vi "field_sweep_agilent_0.vi"() -> ()   [LabVIEW 2016]
uses:
  Controls/Data.ctl
  Controls/State.ctl
  <vilib>/Utility/error.llb/DialogType.ctl
  <vilib>/DAQmx/write.llb/DAQmx Write (Analog DBL 1Chan 1Samp).vi
  <vilib>/DAQmx/create/channels.llb/DAQmx Create Channel (AO-Voltage-Basic).vi
  <vilib>/DAQmx/miscellaneous.llb/DAQmx Fill In Error Info.vi
  <instrlib>/Keysight PNA Series/Keysight PNA Series.lvlib
panel:
  in  "Display Format":i32(ring) items=["Magnitude Linear", "Magnitude Logarithmic", "Phase", "Unwrapped phase", "Imaginary", "Real", "Polar", "Smith Chart", "Smith Admittance", "SWR", "Group Delay", "Kelvin", "Fahrenheit", "Celsius"]
  in  "Data Type":i32(ring) items=["FDATA", "RDATA", "SDATA", "FMEM", "SMEM", "SDIV"]
  in  "Sweep Generation":i32(ring)=1 items=["Stepped", "Analog"]
  in  "IF Bandwidth (Hz)":dbl=1000.0 min=1.0 max=40000.0 step=1.0 format="%#_6p"
  in  "Sweep Mode":i32(ring) items=["Chopped", "Alternate"]
  in  "Sweep Type":i32(ring) items=["Linear", "Logarithmic", "Power", "CW", "Segment", "Phase"]
  out "Analyzer Name Out":refnum<visa-resource-name>
  in  "Analyzer name In":refnum<visa-resource-name>="vna"
  in  "Clear button":bool
  in  "Hysteresis":bool caption="Hysteresis On/Off"
  out "DAQ channel Out":tag="DAQ_6363/ao1"
  in  "Averaging Points":i32=10 min=1 max=3201 step=1
  in  "DAQ channel In":tag="DAQ_6363/ao1"
  in  "Exit Button":bool
  in  "Speed (Oe/sec)":dbl=5.0
  in  "Frequency (Hz)":dbl=3000000000.0 min=10000000.0 max=6000000000.0 format="%#_6p"
  in  "Save Button":bool
  out "Status":string="Initializing..."
  out "Cursor":cluster{"x":dbl, "y":dbl} {"x" format="%.2f"; "y" format="%.5f"}
  out "Error Out":errorcluster={"status"=TRUE, "code"=-1073807346, "source"="VISA Open in Keysight PNA Series.lvlib:Initialize.vi->field_sweep_agilent.vi"}
  in  "Error In (no error)":errorcluster
  out "SpectrumGraph":cluster{"Old Field":dbl[], "Old Signal":dbl[]}[](graph)
  in  "S-parameter":i32(ring)=1 caption="Measurement" items=["S11", "S21"]
  in  "Start Button":bool
  in  "Stop Button":bool
  in  "Output Power (dBm)":dbl=1.0 min=-25.0 max=20.0 step=0.5
  in  "Number of Points":i32=1000 min=1 max=3201 step=1
  in  "Stop H Field (Oe)":dbl=1500.0 min=-6000.0 max=6000.0 format="%#_6f"
  in  "Start H Field (Oe)":dbl=1000.0 min=-6000.0 max=6000.0 format="%#_6f"
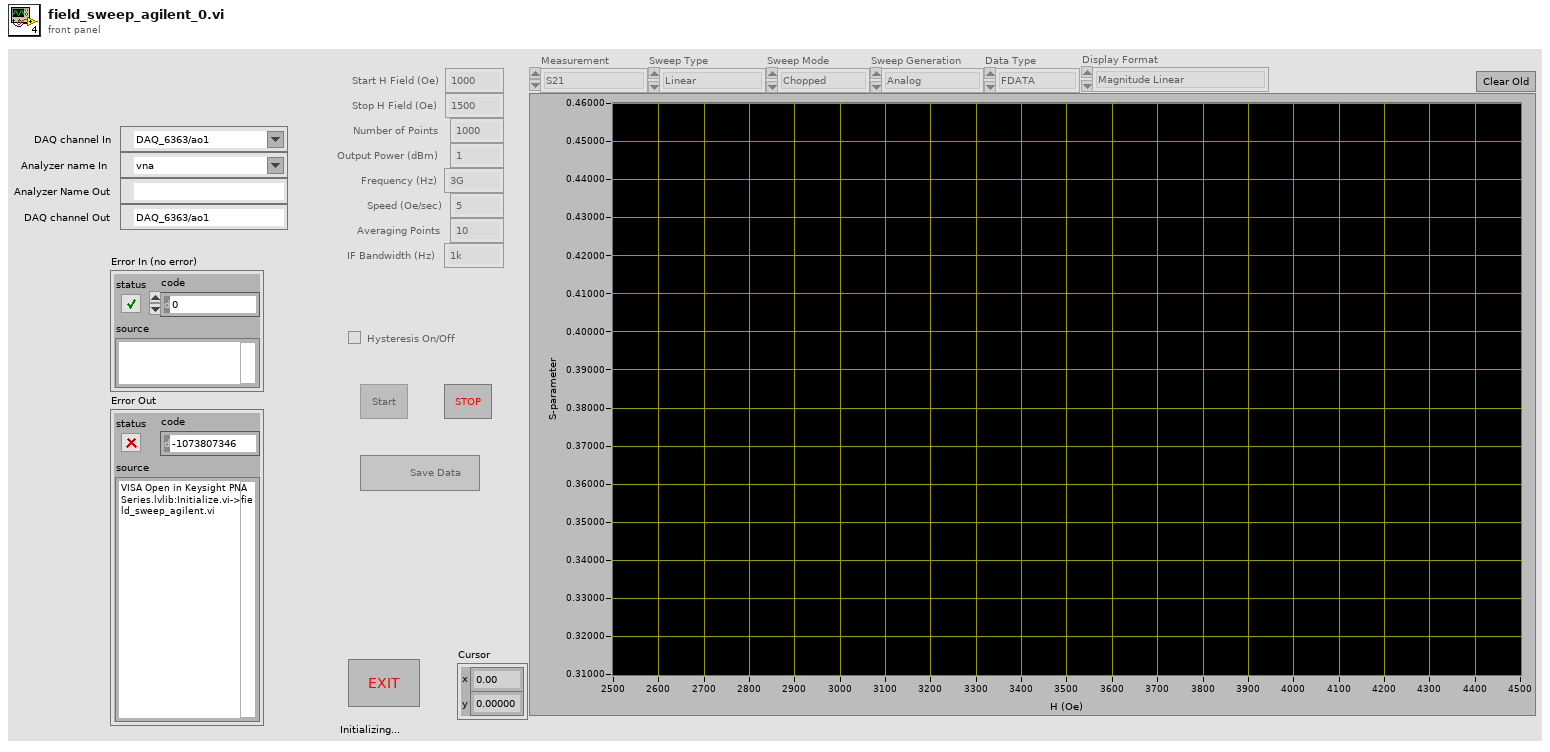
[diagram p1: front panel]
types:
  T1 = typedef "State.ctl" = enum16{"Init", "Idle", "Sweeping up", "Sweeping down", "Running", "Running first time", "Running down", "Shutdown"}
  T2 = typedef "Data.ctl" = cluster{"Field":dbl[], "Signal":dbl[], "Old Field":dbl[], "Old Signal":dbl[]}
  T3 = typedef "DialogType.ctl" = u16
  T4 = typedef "LVPoint32TypeDef.ctl" = cluster{"Horizontal":i32, "Vertical":i32}
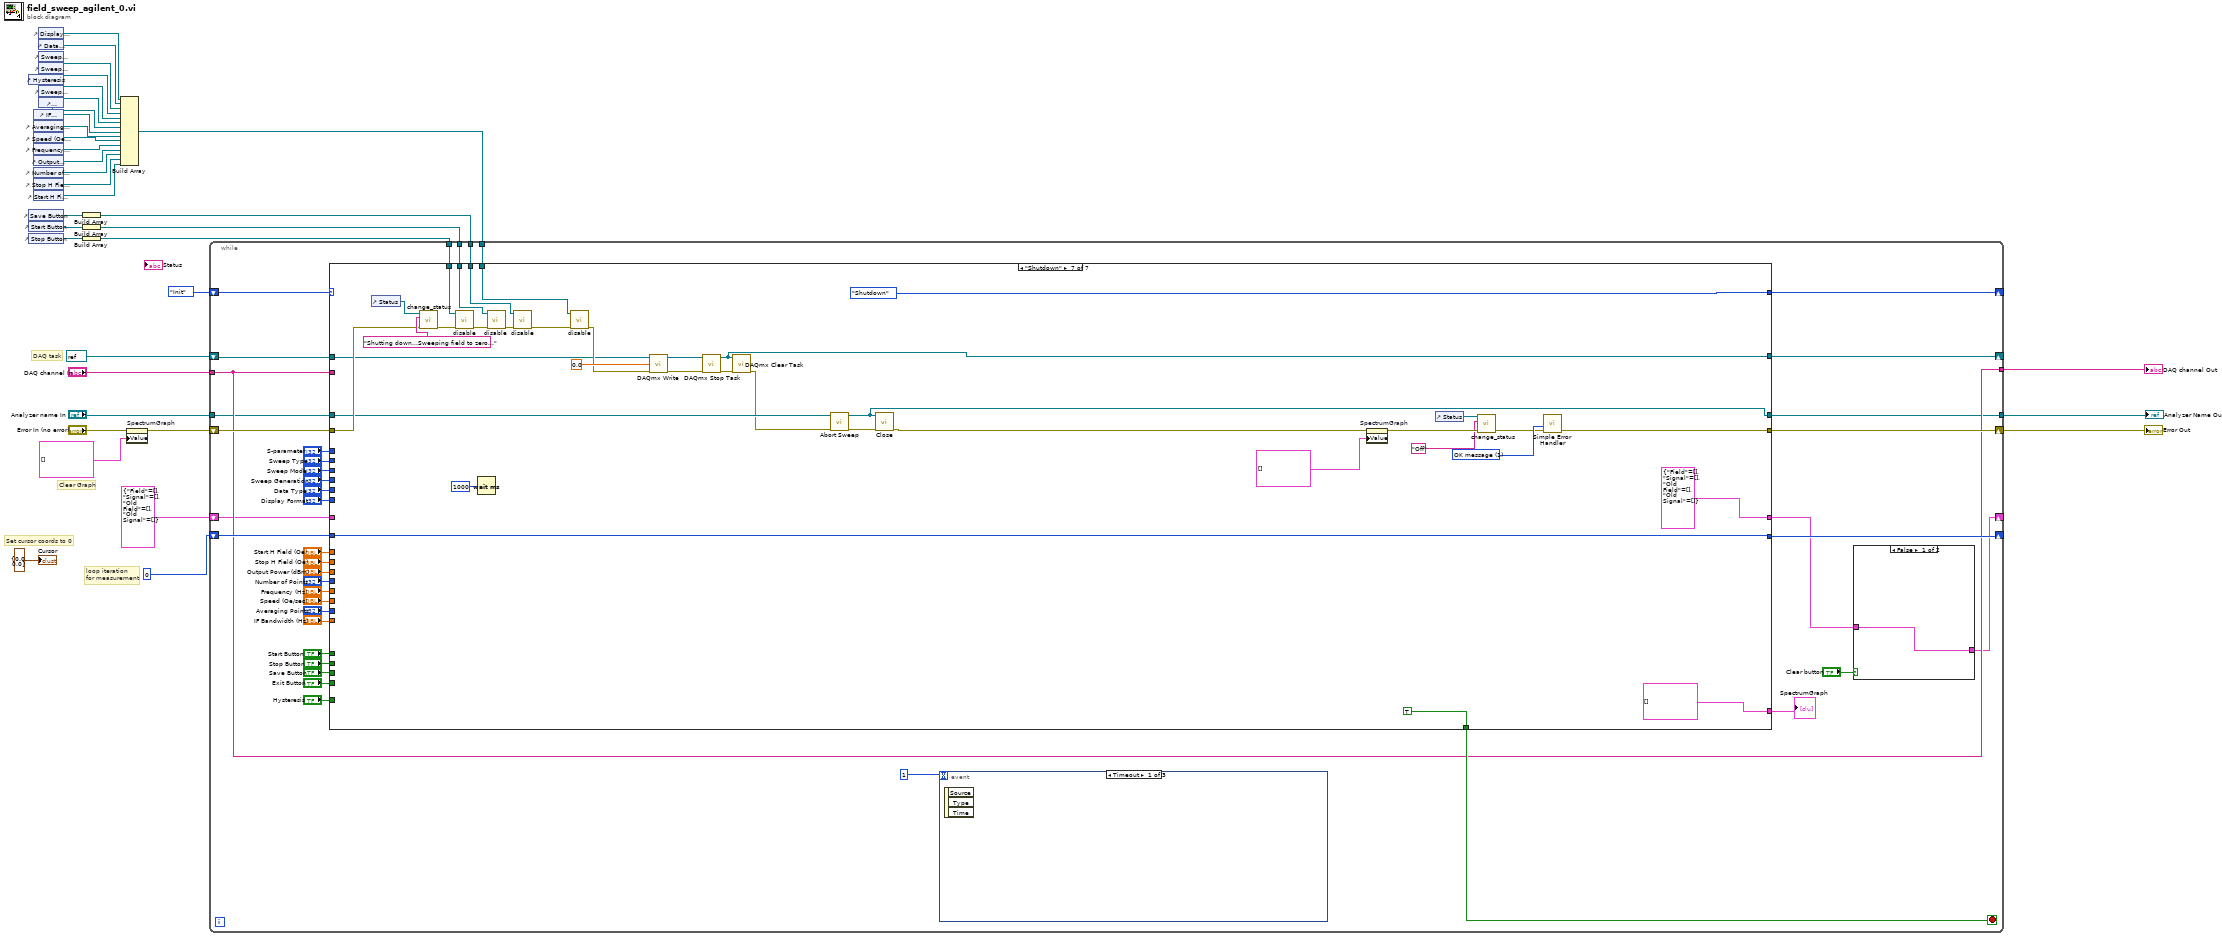
[diagram p0: block diagram]
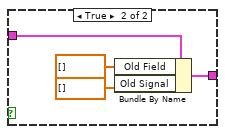
[diagram p2: hidden frame]
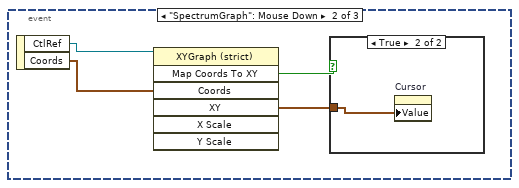
[diagram p3: hidden frame]
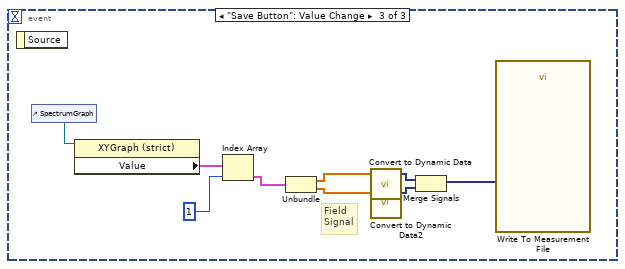
[diagram p5: hidden frame]
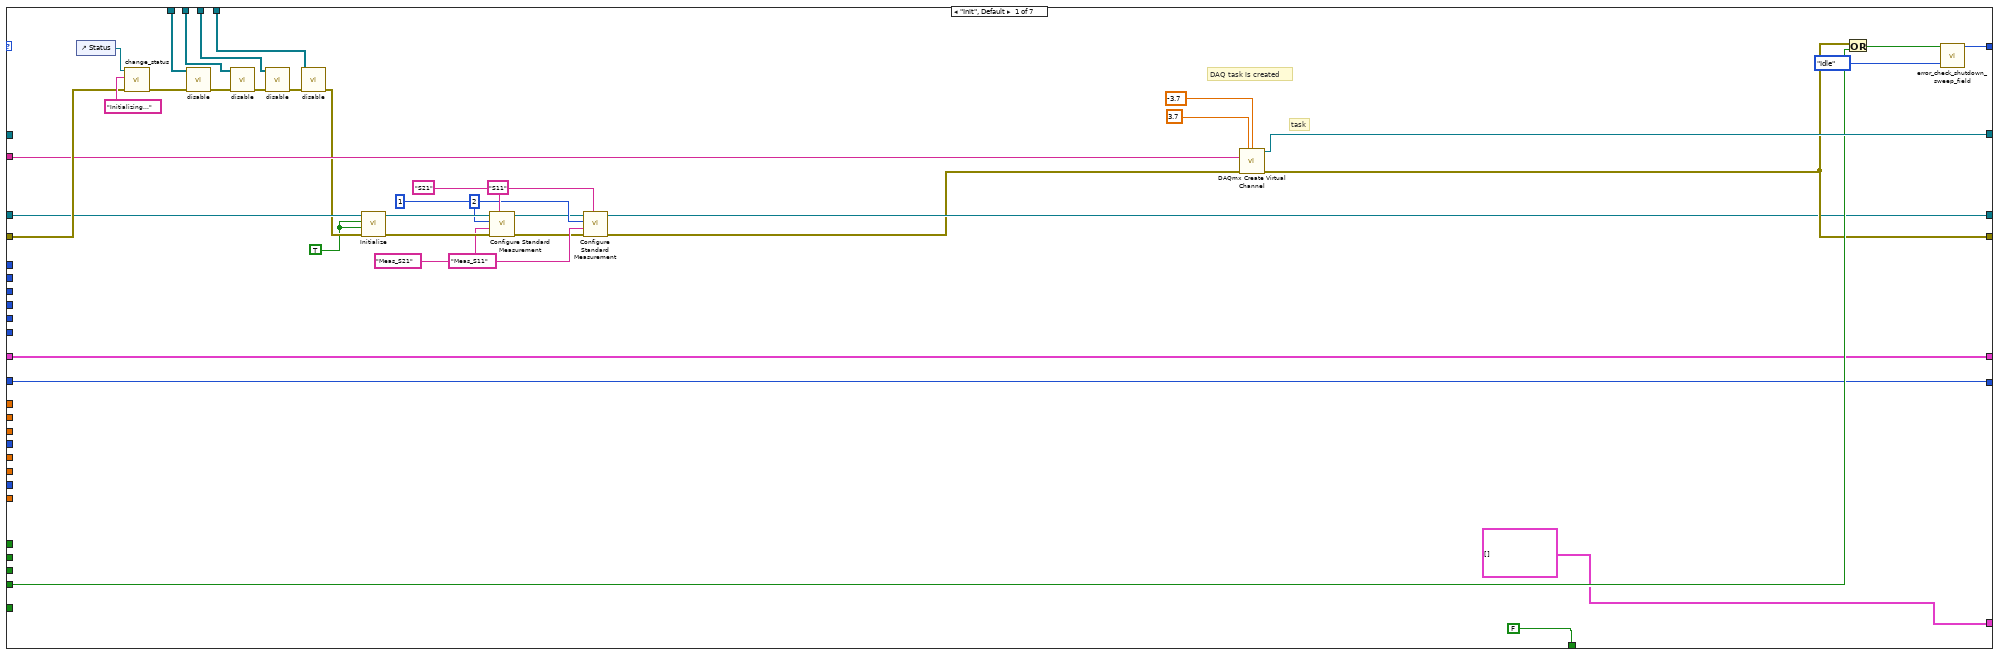
[diagram p6: hidden frame]
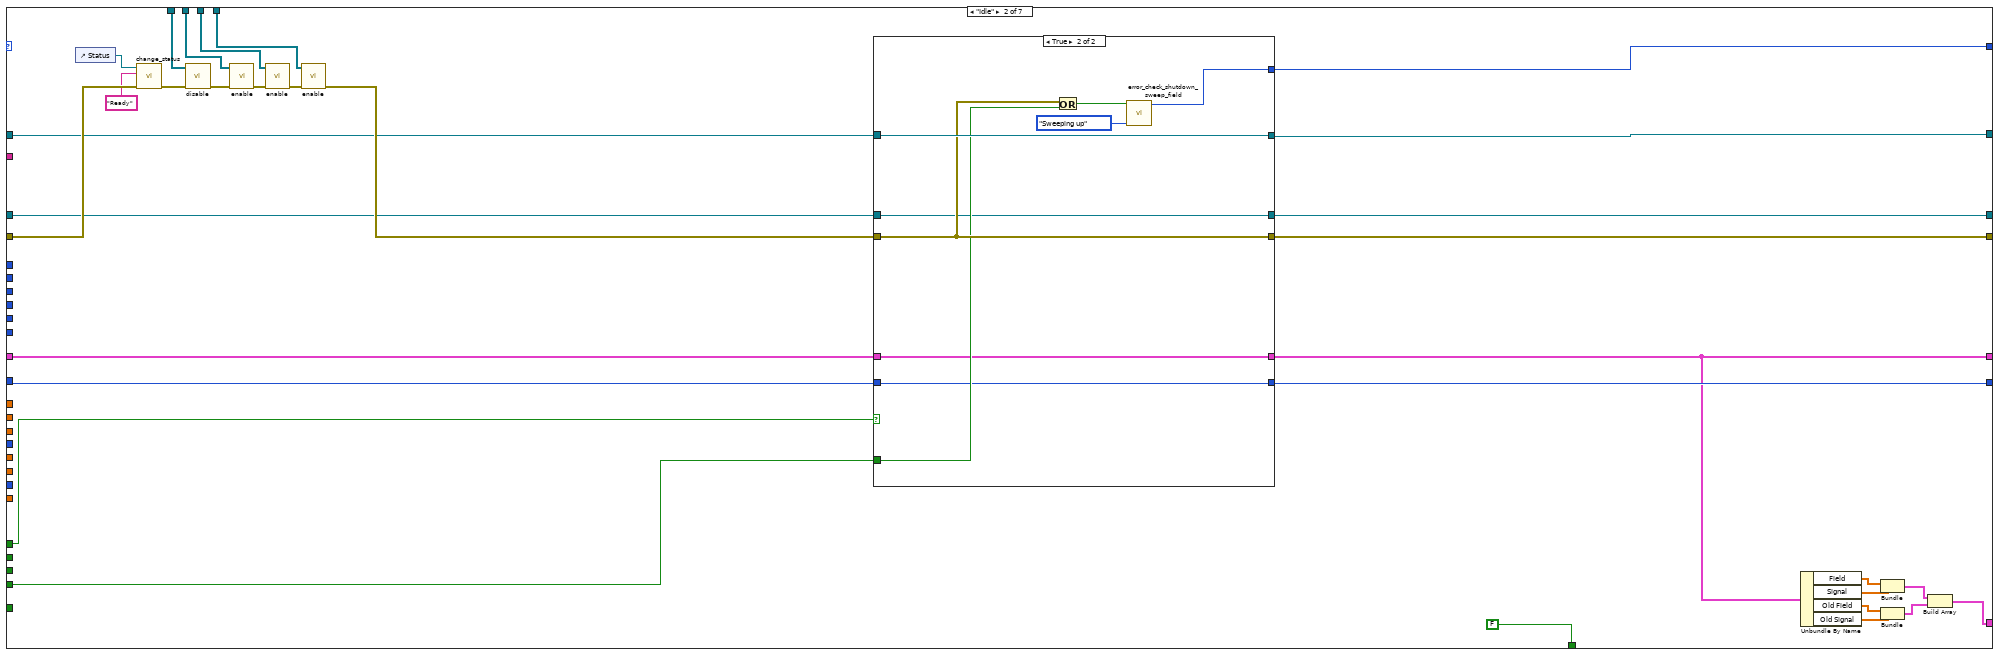
[diagram p7: hidden frame]
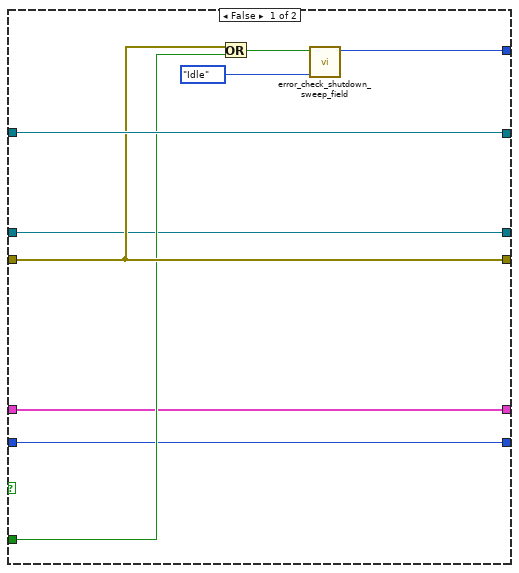
[diagram p8: hidden frame]
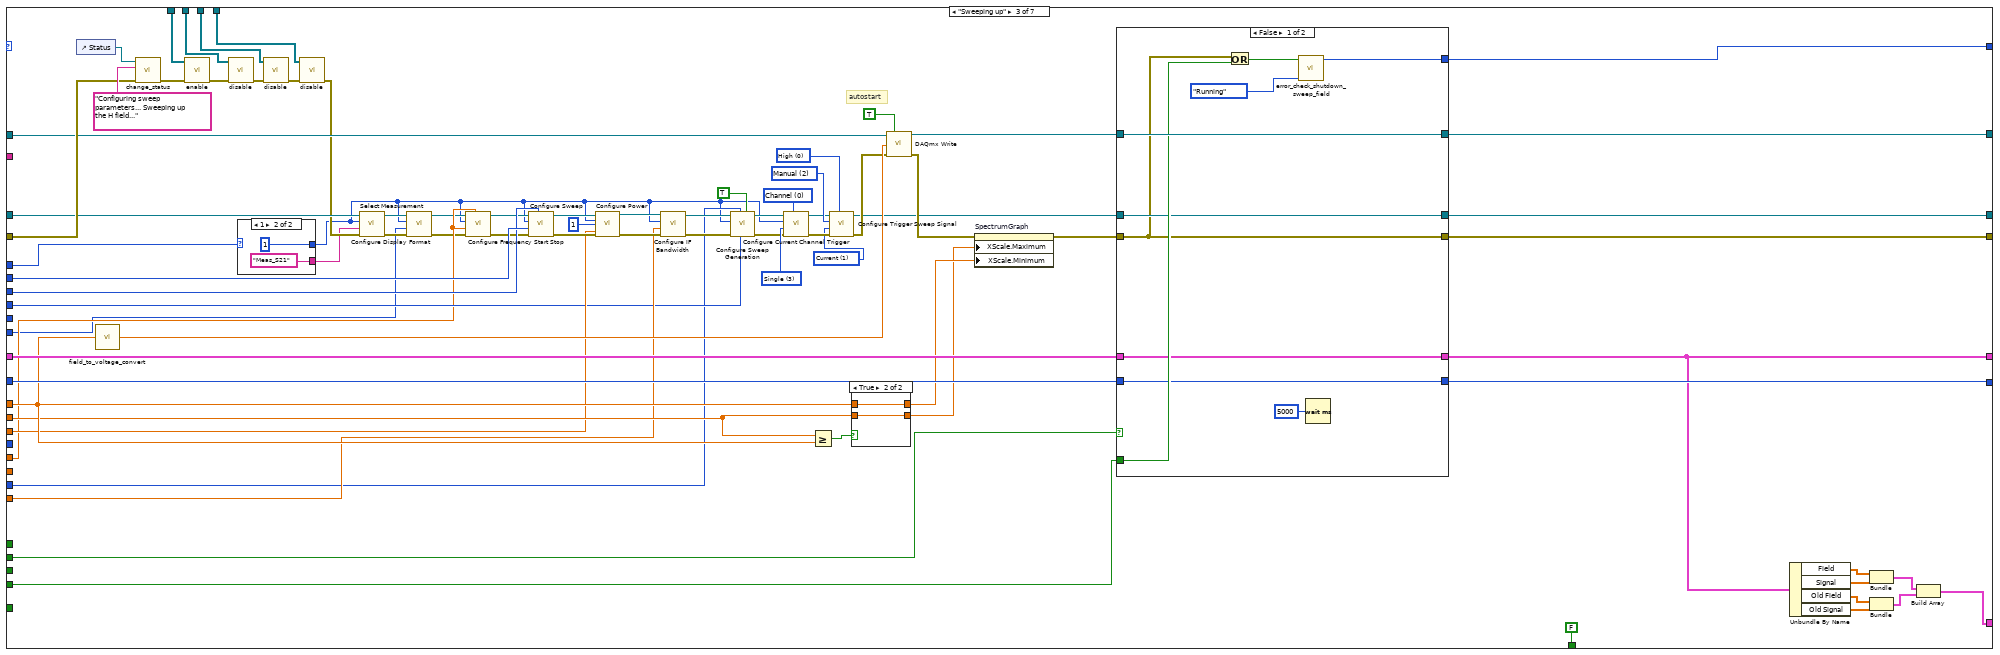
[diagram p9: hidden frame]
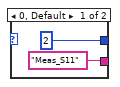
[diagram p10: hidden frame]
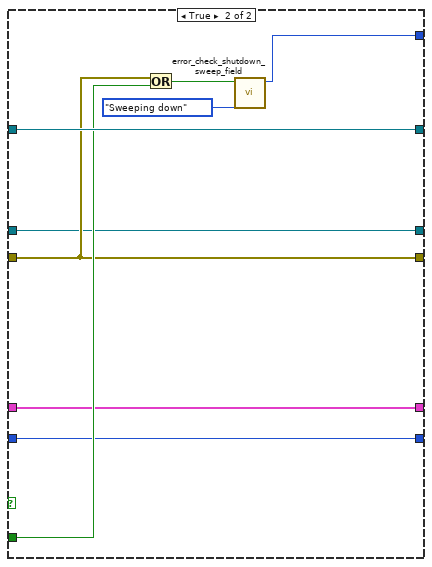
[diagram p12: hidden frame]
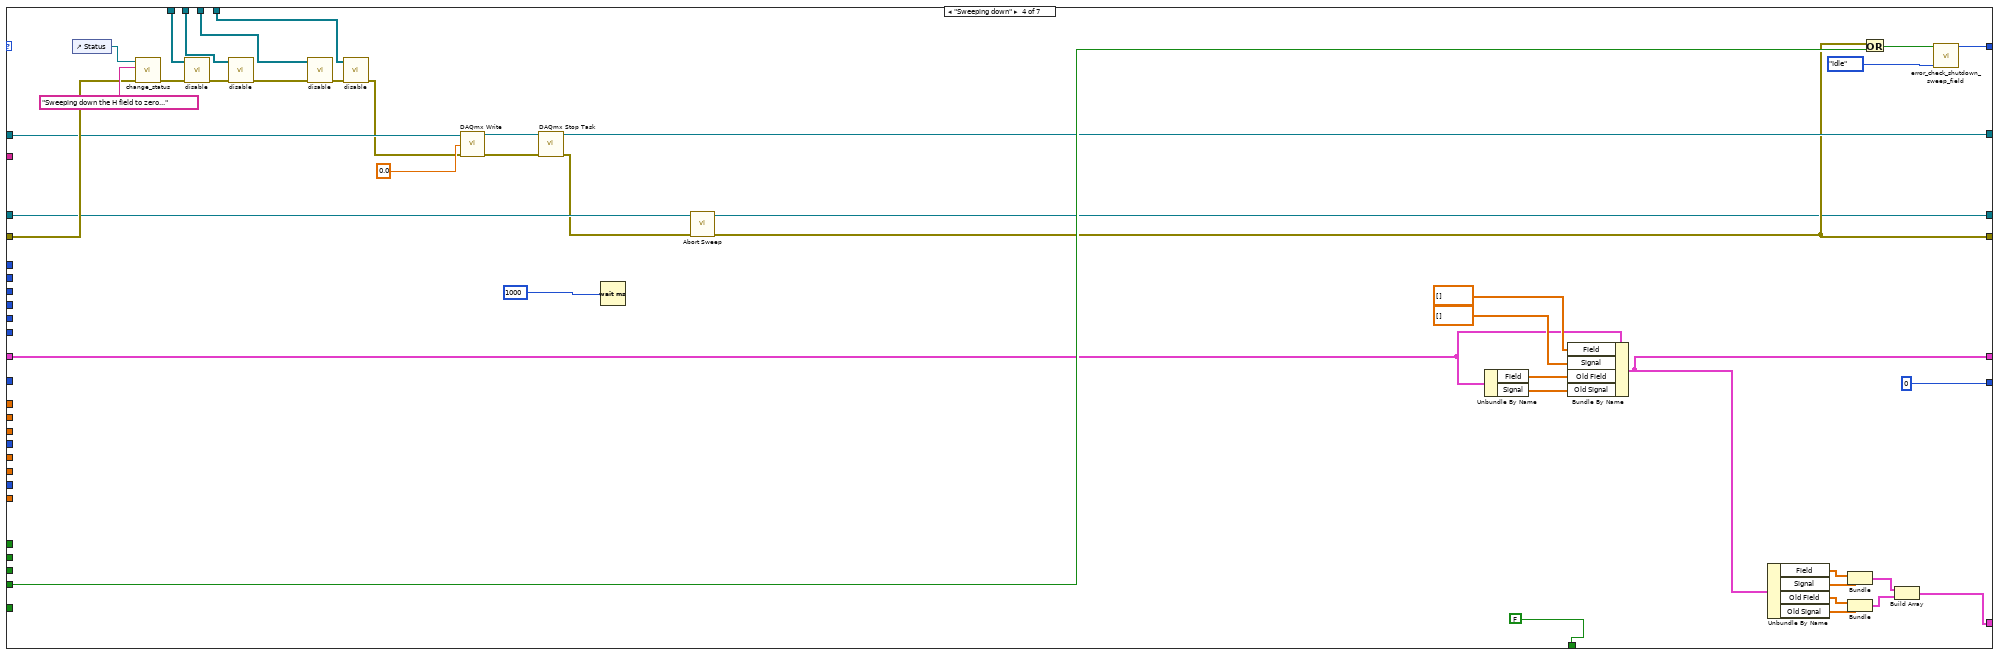
[diagram p13: hidden frame]
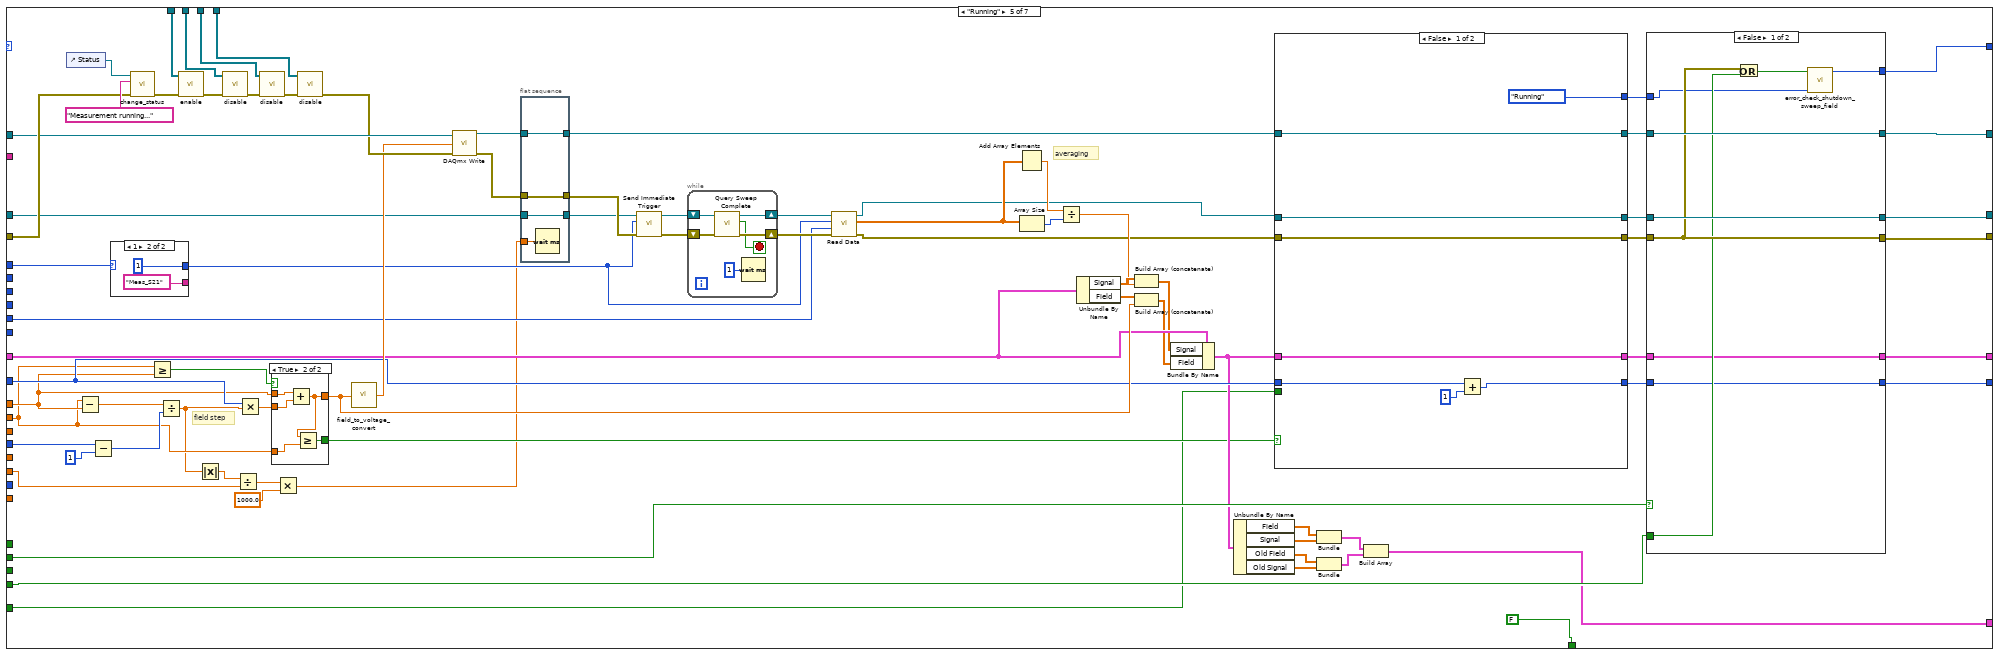
[diagram p14: hidden frame]
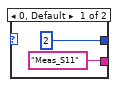
[diagram p15: hidden frame]
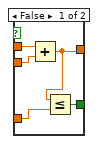
[diagram p16: hidden frame]
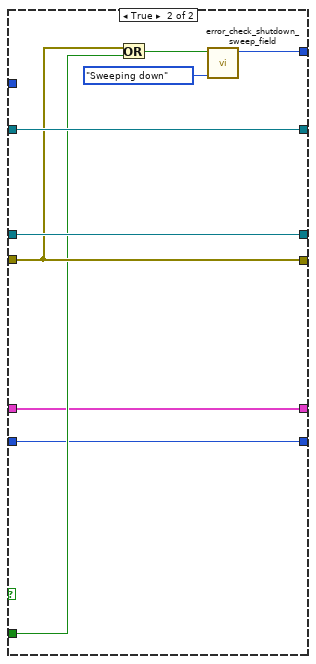
[diagram p17: hidden frame]
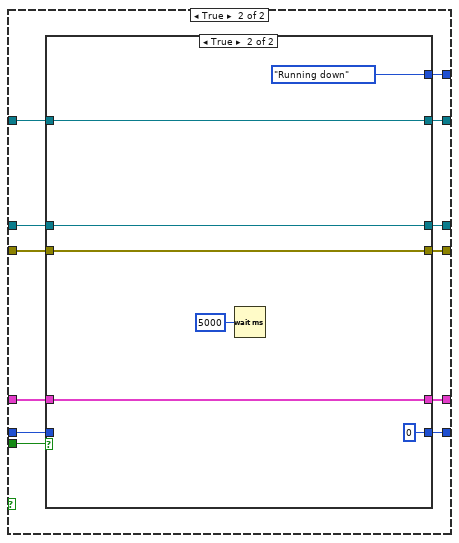
[diagram p18: hidden frame]
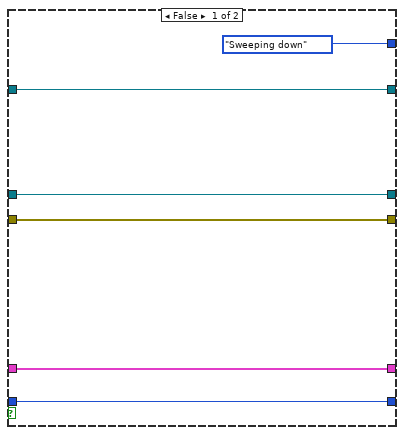
[diagram p19: hidden frame]
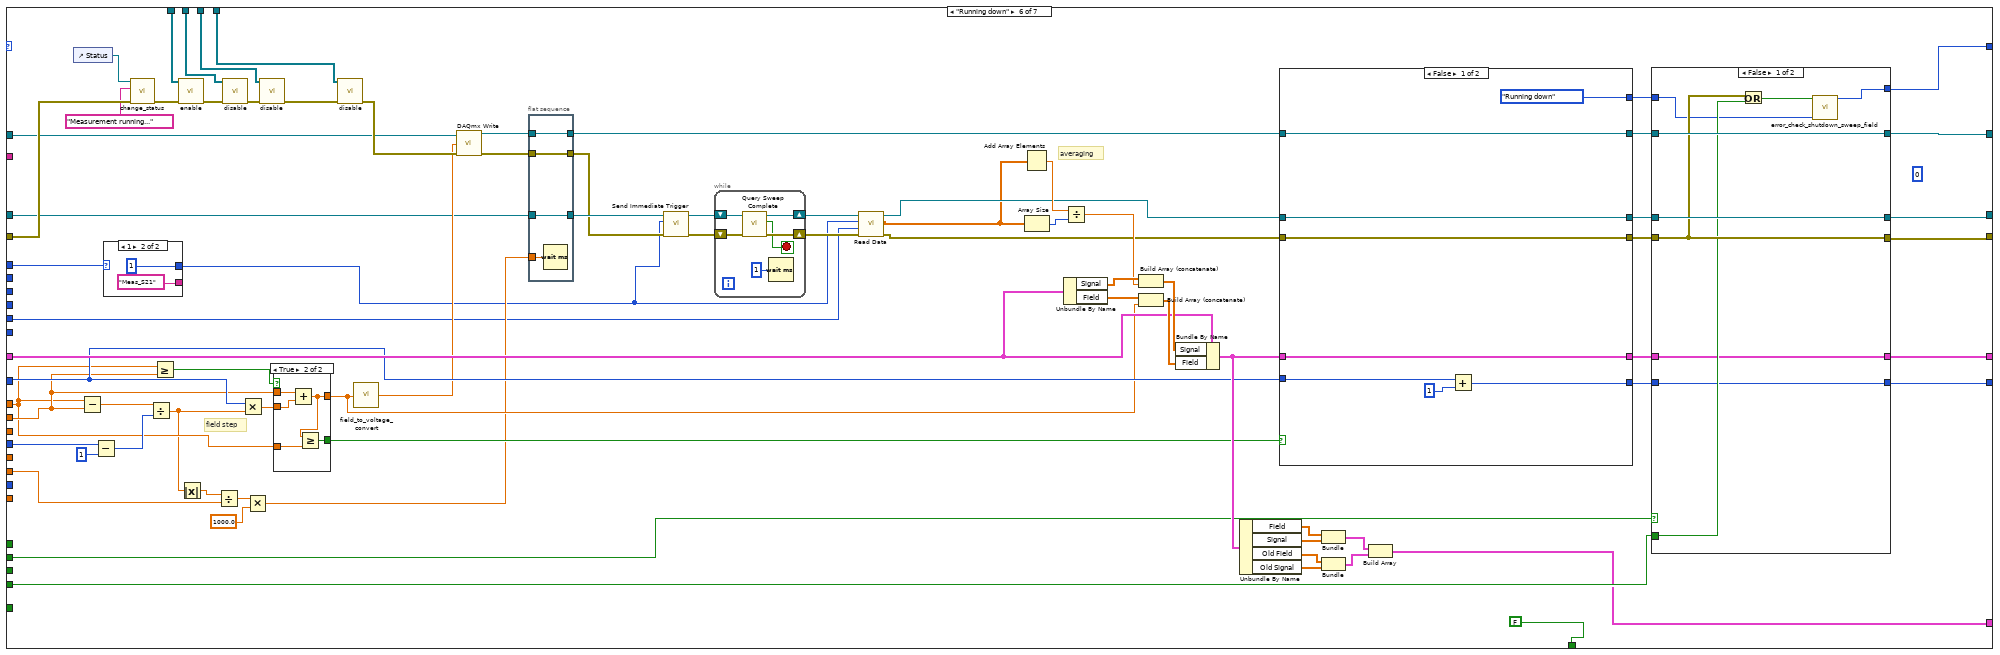
[diagram p20: hidden frame]
diagram:
  # "loop iteration\nfor measurement"
  # "DAQ task"
  # "Set cursor coords to 0"
  # "Clear Graph"
  n1 = control-ref of="Hysteresis"() -> (w10:refnum<vi>)
  n2 = control-ref of="Save Button"() -> (w21:refnum<vi>)
  n3 = control-ref of="Start Button"() -> (w28:refnum<vi>)
  n4 = control-ref of="Stop Button"() -> (w27:refnum<vi>)
  n5 = control-ref of="IF Bandwidth (Hz)"() -> (w4:refnum<vi>)
  n6 = control-ref of="Averaging Points"() -> (w18:refnum<vi>)
  n7 = control-ref of="Speed (Oe/sec)"() -> (w34:refnum<vi>)
  n8 = control-ref of="Frequency (Hz)"() -> (w33:refnum<vi>)
  n9 = control-ref of="Output Power (dBm)"() -> (w32:refnum<vi>)
  n10 = control-ref of="Number of Points"() -> (w31:refnum<vi>)
  n11 = control-ref of="Stop H Field (Oe)"() -> (w30:refnum<vi>)
  n12 = control-ref of="Start H Field (Oe)"() -> (w29:refnum<vi>)
  n13 = control-ref of="Display Format"() -> (w1:refnum<vi>)
  n14 = control-ref of="Data Type"() -> (w3:refnum<vi>)
  n15 = control-ref of="Sweep Generation"() -> (w5:refnum<vi>)
  n16 = control-ref of="Sweep Mode"() -> (w6:refnum<vi>)
  n17 = control-ref of="Sweep Type"() -> (w7:refnum<vi>)
  n18 = control-ref of="S-parameter"() -> (w11:refnum<vi>)
  n19 = Build Array(w21) -> (w20:refnum<vi>[])
  n20 = Build Array(w28) -> (w25:refnum<vi>[])
  n21 = Build Array(w27) -> (w24:refnum<vi>[])
  n22 = Build Array(w1, w3, w5, w6, w10, w7, w11, w4, w18, w34, w33, w32, w31, w30, w29) -> (w26:refnum<vi>[])
  n23 = property on="SpectrumGraph" class="XYGraph (strict)"(error in="Error In (no error)", "Value"=cluster{"Old Field":dbl[], "Old Signal":dbl[]}[] [] ("SpectrumGraph")) -> (error out=w15:errorcluster)  [unwired: 1 in, 1 out]
  n24 = while {
    shift-right: [w73] -> _
    shift-left: State."Init" -> [w37]
    shift-right: [w54] -> _
    shift-left: 0 -> [w56]
    tunnel: w26 -> [w76]
    tunnel: w25 -> [w75]
    tunnel: w24 -> [w74]
    tunnel: "DAQ channel In" -> [w53]
    shift-right: [w72] -> w12
    shift-left: w15 -> [w71]
    shift-right: [w70] -> _
    shift-left: refnum<k21> refnum ("task in") -> [w69]
    tunnel: w20 -> [w68]
    shift-right: [w45] -> _
    shift-left: T2 {"Field"=[], "Signal"=[], "Old Field"=[], "Old Signal"=[]} ("Cluster") -> [w51]
    tunnel: [w53] -> w17
    tunnel: "Analyzer name In" -> [w44]
    tunnel: [w43] -> w8
    stop <- w63 stop-if-true
    n25 = case shown="\"Shutdown\"" w37 {
      tunnel: w76 -> [w122 w163 w254 w321 w401 w552 w645]
      tunnel: w75 -> [w132 w165 w256 w319 w403 w554 w647]
      tunnel: w74 -> [w134 w166 w257 w318 w405 w555 w648]
      tunnel: w71 -> [w128 w158 w252 w325 w399 w558 w643]
      tunnel: [w118 w150 w246 w315 w369 w519 State."Shutdown"] -> w73
      tunnel: w53 -> [w125 _ _ _ _ _ _]
      tunnel: [w117 w153 w250 w291 w375 w521 w640] -> w72
      tunnel: [w124 w151 w249 w310 w378 w520 w641] -> w70
      tunnel: w69 -> [_ w152 w239 w323 w398 w532 w634]
      tunnel: w68 -> [w123 w164 w255 w320 w402 w553 w646]
      tunnel: "Start Button" -> [_ w155 _ _ _ _ _]
      tunnel: "Stop Button" -> [_ _ w251 _ w374 w531 _]
      tunnel: "Save Button" -> [_ _ _ _ _ _ _]
      tunnel: "Exit Button" -> [w119 w149 w245 w316 w373 w524 _]
      tunnel: [FALSE FALSE FALSE FALSE FALSE FALSE TRUE] -> w63
      tunnel: "Start H Field (Oe)" -> [_ _ w236 _ w355 w508 _]
      tunnel: "Stop H Field (Oe)" -> [_ _ w235 _ w353 w509 _]
      tunnel: "Output Power (dBm)" -> [_ _ w211 _ _ _ _]
      tunnel: "Number of Points" -> [_ _ _ _ w390 w512 _]
      tunnel: "Frequency (Hz)" -> [_ _ w201 _ _ _ _]
      tunnel: "Speed (Oe/sec)" -> [_ _ _ _ w391 w501 _]
      tunnel: w56 -> [w115 w147 w244 _ w380 w513 w631]
      tunnel: "Averaging Points" -> [_ _ w204 _ _ _ _]
      tunnel: [w115 w148 w243 0 w371 w522 w631] -> w54
      tunnel: [w113 w137 w225 w294 w363 w523 T2 {"Field"=[], "Signal"=[], "Old Field"=[], "Old Signal"=[]} ("Cluster")] -> w46
      tunnel: w51 -> [w113 w145 w240 w305 w367 w530 _]
      tunnel: "Hysteresis" -> [_ _ _ _ w351 _ _]
      tunnel: "S-parameter" -> [_ _ w222 _ w345 w489 _]
      tunnel: [cluster{"Old Field":dbl[], "Old Signal":dbl[]}[] [] w138 w226 w295 w350 w507 cluster{"Old Field":dbl[], "Old Signal":dbl[]}[] []] -> w48
      tunnel: w44 -> [w110 w136 w224 w293 w343 w498 w622]
      tunnel: [w97 w135 w205 w290 w334 w497 w619] -> w43
      tunnel: "Sweep Type" -> [_ _ w220 _ _ _ _]
      tunnel: "Sweep Mode" -> [_ _ w219 _ _ _ _]
      tunnel: "IF Bandwidth (Hz)" -> [_ _ w210 _ _ _ _]
      tunnel: "Sweep Generation" -> [_ _ w209 _ _ _ _]
      tunnel: "Data Type" -> [_ _ _ _ w332 w487 _]
      tunnel: "Display Format" -> [_ _ w185 _ _ _ _]
      frame "Init", Default {
        w108 = TRUE ("ID Query (True)")
        # "task"
        # "DAQ task is created"
        n26 = control-ref of="Status"() -> (w130:refnum<vi>)
        n27 = call "change_status.vi"("error in (no error)"=w128, "String"="Initializing...", "String in"=w130) -> ("error out"=w131:errorcluster)  [unwired: 8 in]
        n28 = call "disable.vi"("error in (no error)"=w131, "Array"=w134) -> ("error out"=w133:errorcluster)  [unwired: 9 in]
        n29 = call "disable.vi"("error in (no error)"=w133, "Array"=w132) -> ("error out"=w121:errorcluster)  [unwired: 9 in]
        n30 = call "disable.vi"("error in (no error)"=w121, "Array"=w123) -> ("error out"=w120:errorcluster)  [unwired: 9 in]
        n31 = call "disable.vi"("error in (no error)"=w120, "Array"=w122) -> ("error out"=w109:errorcluster)  [unwired: 9 in]
        n32 = call <instrlib>:"Initialize.vi"("error in (no error)"=w109, "Reset (True)"=w108, "ID Query (True)"=w108, "VISA resource name"=w110) -> ("error out"=w107:errorcluster, "VISA resource name out"=w106:refnum<visa-resource-name>)  [unwired: 6 in]
        n33 = call <instrlib>:"Configure Standard Measurement.vi"("Measurement Parameters (S11)"="S21", "error in (no error)"=w107, "Measurement Name (CH1_S11_1)"="Meas_S21", "Channel (1)"=1, "VISA resource name"=w106) -> ("error out"=w99:errorcluster, "VISA resource name out"=w98:refnum<visa-resource-name>)  [unwired: 5 in]
        n34 = call <instrlib>:"Configure Standard Measurement.vi"("Measurement Parameters (S11)"="S11", "error in (no error)"=w99, "Measurement Name (CH1_S11_1)"="Meas_S11", "Channel (1)"=2, "VISA resource name"=w98) -> ("error out"=w96:errorcluster, "VISA resource name out"=w97:refnum<visa-resource-name>)  [unwired: 5 in]
        n35 = call-poly <vilib>:"DAQmx Create Virtual Channel.vi"("maximum value"=3.7, "minimum value"=-3.7, "physical channels"=w125, "error in"=w96) -> ("task out"=w124:refnum<k21>, "error out"=w117:errorcluster)  [unwired: 10 in]
        n36 = Or(x=w117, y=w119) -> (x .or. y?=w116:bool)
        n37 = call "error_check_shutdown_sweep_field.vi"("State In"=State."Idle", "Boolean"=w116) -> ("State Out"=w118:T1)  [unwired: 9 in]
      }
      frame "Idle" {
        n38 = control-ref of="Status"() -> (w157:refnum<vi>)
        n39 = call "change_status.vi"("error in (no error)"=w158, "String"="Ready", "String in"=w157) -> ("error out"=w159:errorcluster)  [unwired: 8 in]
        n40 = call "disable.vi"("error in (no error)"=w159, "Array"=w166) -> ("error out"=w162:errorcluster)  [unwired: 9 in]
        n41 = call "enable.vi"("error in (no error)"=w162, "Array"=w165) -> ("error out"=w161:errorcluster)  [unwired: 9 in]
        n42 = call "enable.vi"("error in (no error)"=w161, "Array"=w164) -> ("error out"=w160:errorcluster)  [unwired: 9 in]
        n43 = call "enable.vi"("error in (no error)"=w160, "Array"=w163) -> ("error out"=w154:errorcluster)  [unwired: 9 in]
        n44 = case shown="True" w155 {
          tunnel: w154 -> [w172 w182]
          tunnel: [w172 w182] -> w153
          tunnel: w152 -> [w175 w184]
          tunnel: [w175 w184] -> w151
          tunnel: [w173 w180] -> w150
          tunnel: w149 -> [w171 w181]
          tunnel: [w170 w179] -> w148
          tunnel: w147 -> [w170 w179]
          tunnel: w145 -> [w169 w178]
          tunnel: [w169 w178] -> w137
          tunnel: w136 -> [w167 w176]
          tunnel: [w167 w176] -> w135
          frame False {
            n45 = Or(x=w172, y=w171) -> (x .or. y?=w174:bool)
            n46 = call "error_check_shutdown_sweep_field.vi"("State In"=State."Idle", "Boolean"=w174) -> ("State Out"=w173:T1)  [unwired: 9 in]
          }
          frame True {
            n47 = Or(x=w182, y=w181) -> (x .or. y?=w183:bool)
            n48 = call "error_check_shutdown_sweep_field.vi"("State In"=State."Sweeping up", "Boolean"=w183) -> ("State Out"=w180:T1)  [unwired: 9 in]
          }
        }
        n49 = Unbundle By Name(w137) -> ("Field"=w144:dbl[], "Signal"=w143:dbl[], "Old Field"=w142:dbl[], "Old Signal"=w141:dbl[])
        n50 = Bundle("Field"=w144, "Signal"=w143) -> (w140:cluster{"Field":dbl[], "Signal":dbl[]})  [unwired: 1 in]
        n51 = Bundle("Old Field"=w142, "Old Signal"=w141) -> (w139:cluster{"Old Field":dbl[], "Old Signal":dbl[]})  [unwired: 1 in]
        n52 = Build Array(w140, w139) -> (w138:cluster{"Old Field":dbl[], "Old Signal":dbl[]}[])
      }
      frame "Sweeping up" {
        w193 = 0 items=["High", "Low"] ("Trigger Level (1: Low)")
        w194 = 1 items=["All", "Current"] ("Trigger Scope (0: All)")
        w195 = 0 items=["Channel", "Sweep", "Point", "Trace"] ("Trigger Mode (0: Channel)")
        w200 = 3 items=["Hold", "Continuous", "Groups", "Single"] ("Trigger Condition (1: Continuous)")
        w207 = 2 items=["Immediate", "External", "Manual"] ("Trigger Source (0: Immediate)")
        # "autostart"
        n53 = control-ref of="Status"() -> (w253:refnum<vi>)
        n54 = call "field_to_voltage_convert.vi"("Start H Field (Oe)"=w236) -> ("Numeric"=w247:dbl)
        n55 = call "change_status.vi"("error in (no error)"=w252, "String"="Configuring sweep parameters... Sweeping up the H field...", "String in"=w253) -> ("error out"=w261:errorcluster)  [unwired: 8 in]
        n56 = call "enable.vi"("error in (no error)"=w261, "Array"=w257) -> ("error out"=w260:errorcluster)  [unwired: 9 in]
        n57 = call "disable.vi"("error in (no error)"=w260, "Array"=w256) -> ("error out"=w259:errorcluster)  [unwired: 9 in]
        n58 = case shown="1" w222 {
          tunnel: [2 ("Channel (1)") 1 ("Channel (1)")] -> w186
          tunnel: ["Meas_S11" ("Measurement Name (CH1_S11_1)") "Meas_S21" ("Measurement Name (CH1_S11_1)")] -> w221
          frame 0, Default {
          }
          frame 1 {
          }
        }
        n59 = call "disable.vi"("error in (no error)"=w259, "Array"=w255) -> ("error out"=w258:errorcluster)  [unwired: 9 in]
        n60 = call "disable.vi"("error in (no error)"=w258, "Array"=w254) -> ("error out"=w223:errorcluster)  [unwired: 9 in]
        n61 = call <instrlib>:"Select Measurement.vi"("error in (no error)"=w223, "Measurement Name (CH1_S11_1)"=w221, "Channel (1)"=w186, "VISA resource name"=w224) -> ("error out"=w190:errorcluster, "VISA resource name out"=w189:refnum<visa-resource-name>)  [unwired: 6 in]
        n62 = call <instrlib>:"Configure Display Format.vi"("error in (no error)"=w190, "Display Format (0: Magnitude Linear)"=w185, "Channel (1)"=w186, "VISA resource name"=w189) -> ("error out"=w187:errorcluster, "VISA resource name out"=w188:refnum<visa-resource-name>)  [unwired: 6 in]
        n63 = call <instrlib>:"Configure Frequency Start Stop.vi"("Stop Frequency (2E+6 Hz)"=w201, "error in (no error)"=w187, "Start Frequency (1E+6 Hz)"=w201, "Channel (1)"=w186, "VISA resource name"=w188) -> ("error out"=w203:errorcluster, "VISA resource name out"=w202:refnum<visa-resource-name>)  [unwired: 5 in]
        n64 = call <instrlib>:"Configure Sweep.vi"("Sweep Mode (0: Chopped)"=w219, "error in (no error)"=w203, "Sweep Type (0: Linear)"=w220, "Channel (1)"=w186, "VISA resource name"=w202) -> ("error out"=w218:errorcluster, "VISA resource name out"=w216:refnum<visa-resource-name>)  [unwired: 5 in]
        n65 = call <instrlib>:"Configure Power.vi"("VISA resource name"=w216, "Channel (1)"=w186, "Port (1)"=1, "error in (no error)"=w218, "Power Level (0 dBm)"=w211) -> ("VISA resource name out"=w215:refnum<visa-resource-name>, "error out"=w217:errorcluster)  [unwired: 9 in]
        n66 = call <instrlib>:"Configure IF Bandwidth.vi"("error in (no error)"=w217, "Bandwidth (100000 Hz)"=w210, "Channel (1)"=w186, "VISA resource name"=w215) -> ("error out"=w213:errorcluster, "VISA resource name out"=w214:refnum<visa-resource-name>)  [unwired: 6 in]
        n67 = call <instrlib>:"Configure Sweep Generation.vi"("Auto Sweep or Dwell Time (T: Enable)"=TRUE, "Sweep Generation (1: Analog)"=w209, "Sweep Points (201)"=w204, "error in (no error)"=w213, "Channel (1)"=w186, "VISA resource name"=w214) -> ("error out"=w199:errorcluster, "VISA resource name out"=w197:refnum<visa-resource-name>)  [unwired: 4 in]
        n68 = call <instrlib>:"Configure Current Channel Trigger.vi"("Trigger Mode (0: Channel)"=w195, "error in (no error)"=w199, "Trigger Condition (1: Continuous)"=w200, "Channel (1)"=w186, "VISA resource name"=w197) -> ("error out"=w198:errorcluster, "VISA resource name out"=w196:refnum<visa-resource-name>)  [unwired: 5 in]
        n69 = Greater Or Equal?(x=w235, y=w236) -> (x >= y?=w237:bool)
        n70 = call <instrlib>:"Configure Trigger Sweep Signal.vi"("Trigger Level (1: Low)"=w193, "error in (no error)"=w198, "Trigger Scope (0: All)"=w194, "Trigger Source (0: Immediate)"=w207, "VISA resource name"=w196) -> ("error out"=w206:errorcluster, "VISA resource name out"=w192:refnum<visa-resource-name>)  [unwired: 5 in]
        n71 = case shown="True" w237 {
          tunnel: w236 -> [w268 w270]
          tunnel: w235 -> [w267 w269]
          tunnel: [w267 w270] -> w234
          tunnel: [w268 w269] -> w233
          frame False {
          }
          frame True {
          }
        }
        n72 = call-poly <vilib>:"DAQmx Write.vi"("task/channels in"=w239, "auto start"=TRUE, "data"=w247, "error in"=w206) -> ("task out"=w248:refnum<k21>, "error out"=w241:errorcluster)  [unwired: 9 in, 1 out]
        n73 = property on="SpectrumGraph" class="XYGraph (strict)"(error in=w241, "XScale.Maximum"=w233, "XScale.Minimum"=w234) -> (error out=w191:errorcluster)  [unwired: 1 in, 1 out]
        n74 = case shown="False" w251 {
          tunnel: w191 -> [w271 w285]
          tunnel: w248 -> [w280 w289]
          tunnel: [w271 w285] -> w250
          tunnel: [w280 w289] -> w249
          tunnel: [w278 w287] -> w246
          tunnel: w245 -> [w277 w286]
          tunnel: w244 -> [w275 w284]
          tunnel: [w275 w284] -> w243
          tunnel: w240 -> [w274 w283]
          tunnel: [w274 w283] -> w225
          tunnel: w192 -> [w272 w281]
          tunnel: [w272 w281] -> w205
          frame False {
            n75 = Or(x=w271, y=w277) -> (x .or. y?=w279:bool)
            n76 = call "error_check_shutdown_sweep_field.vi"("State In"=State."Running", "Boolean"=w279) -> ("State Out"=w278:T1)  [unwired: 9 in]
            n77 = Wait (ms)(milliseconds to wait=u32 5000) -> ()  [unwired: 1 out]
          }
          frame True {
            n78 = Or(x=w285, y=w286) -> (x .or. y?=w288:bool)
            n79 = call "error_check_shutdown_sweep_field.vi"("State In"=State."Sweeping down", "Boolean"=w288) -> ("State Out"=w287:T1)  [unwired: 9 in]
          }
        }
        n80 = Unbundle By Name(w225) -> ("Field"=w232:dbl[], "Signal"=w231:dbl[], "Old Field"=w230:dbl[], "Old Signal"=w229:dbl[])
        n81 = Bundle("Field"=w232, "Signal"=w231) -> (w228:cluster{"Field":dbl[], "Signal":dbl[]})  [unwired: 1 in]
        n82 = Bundle("Old Field"=w230, "Old Signal"=w229) -> (w227:cluster{"Old Field":dbl[], "Old Signal":dbl[]})  [unwired: 1 in]
        n83 = Build Array(w228, w227) -> (w226:cluster{"Old Field":dbl[], "Old Signal":dbl[]}[])
      }
      frame "Sweeping down" {
        n84 = control-ref of="Status"() -> (w314:refnum<vi>)
        n85 = call "change_status.vi"("error in (no error)"=w325, "String"="Sweeping down the H field to zero...", "String in"=w314) -> ("error out"=w329:errorcluster)  [unwired: 8 in]
        n86 = call "disable.vi"("error in (no error)"=w329, "Array"=w318) -> ("error out"=w328:errorcluster)  [unwired: 9 in]
        n87 = call "disable.vi"("error in (no error)"=w328, "Array"=w319) -> ("error out"=w327:errorcluster)  [unwired: 9 in]
        n88 = call "disable.vi"("error in (no error)"=w327, "Array"=w320) -> ("error out"=w326:errorcluster)  [unwired: 9 in]
        n89 = call "disable.vi"("error in (no error)"=w326, "Array"=w321) -> ("error out"=w322:errorcluster)  [unwired: 9 in]
        n90 = call-poly <vilib>:"DAQmx Write.vi"("task/channels in"=w323, "data"=0.0, "error in"=w322) -> ("task out"=w311:refnum<k21>, "error out"=w309:errorcluster)  [unwired: 10 in, 1 out]
        n91 = call <vilib>:"DAQmx Stop Task.vi"("task/channels in"=w311, "error in"=w309) -> ("task out"=w310:refnum<k21>, "error out"=w292:errorcluster)  [unwired: 12 in]
        n92 = Wait (ms)(milliseconds to wait=u32 1000) -> ()  [unwired: 1 out]
        n93 = call <instrlib>:"Abort Sweep.vi"("error in (no error)"=w292, "VISA resource name"=w293) -> ("error out"=w291:errorcluster, "VISA resource name out"=w290:refnum<visa-resource-name>)  [unwired: 8 in]
        n94 = Unbundle By Name(w305) -> ("Field"=w304:dbl[], "Signal"=w303:dbl[])
        n95 = Bundle By Name(cluster=w305, "Field"=dbl[] [], "Signal"=dbl[] [], "Old Field"=w304, "Old Signal"=w303) -> (w294:T2)
        n96 = Unbundle By Name(w294) -> ("Field"=w301:dbl[], "Signal"=w300:dbl[], "Old Field"=w299:dbl[], "Old Signal"=w298:dbl[])
        n97 = Bundle("Field"=w301, "Signal"=w300) -> (w297:cluster{"Field":dbl[], "Signal":dbl[]})  [unwired: 1 in]
        n98 = Bundle("Old Field"=w299, "Old Signal"=w298) -> (w296:cluster{"Old Field":dbl[], "Old Signal":dbl[]})  [unwired: 1 in]
        n99 = Or(x=w291, y=w316) -> (x .or. y?=w317:bool)
        n100 = Build Array(w297, w296) -> (w295:cluster{"Old Field":dbl[], "Old Signal":dbl[]}[])
        n101 = call "error_check_shutdown_sweep_field.vi"("State In"=State."Idle", "Boolean"=w317) -> ("State Out"=w315:T1)  [unwired: 9 in]
      }
      frame "Running" {
        # "averaging"
        # "field step"
        n102 = control-ref of="Status"() -> (w400:refnum<vi>)
        n103 = Subtract(x=w353, y=w355) -> (x-y=w386:dbl)
        n104 = Subtract(x=w390, y=1) -> (x-y=w395:i32)
        n105 = case shown="1" w345 {
          tunnel: [2 ("Channel (1)") 1 ("Channel (1)")] -> w333
          tunnel: ["Meas_S11" ("Measurement Name (CH1_S11_1)") "Meas_S21" ("Measurement Name (CH1_S11_1)")] -> _
          frame 0, Default {
          }
          frame 1 {
          }
        }
        n106 = call "change_status.vi"("error in (no error)"=w399, "String"="Measurement running...", "String in"=w400) -> ("error out"=w406:errorcluster)  [unwired: 8 in]
        n107 = Greater Or Equal?(x=w353, y=w355) -> (x >= y?=w354:bool)
        n108 = Divide(x=w386, y=w395) -> (x/y=w347:dbl)
        n109 = call "enable.vi"("error in (no error)"=w406, "Array"=w405) -> ("error out"=w409:errorcluster)  [unwired: 9 in]
        n110 = Absolute Value(x=w347) -> (abs(x)=w346:dbl)
        n111 = call "disable.vi"("error in (no error)"=w409, "Array"=w403) -> ("error out"=w408:errorcluster)  [unwired: 9 in]
        n112 = Divide(x=w346, y=w391) -> (x/y=w349:dbl)
        n113 = Multiply(x=w380, y=w347) -> (x*y=w394:dbl)
        n114 = call "disable.vi"("error in (no error)"=w408, "Array"=w402) -> ("error out"=w407:errorcluster)  [unwired: 9 in]
        n115 = case shown="True" w354 {
          tunnel: w394 -> [w423 w429]
          tunnel: w355 -> [w424 w428]
          tunnel: [w421 w426] -> w382
          tunnel: w353 -> [w422 w425]
          tunnel: [w420 w427] -> w352
          frame False {
            n116 = Add(x=w424, y=w423) -> (x+y=w421:dbl)
            n117 = Less Or Equal?(x=w421, y=w422) -> (x <= y?=w420:bool)
          }
          frame True {
            n118 = Add(x=w428, y=w429) -> (x+y=w426:dbl)
            n119 = Greater Or Equal?(x=w426, y=w425) -> (x >= y?=w427:bool)
          }
        }
        n120 = Multiply(x=w349, y=1000.0) -> (x*y=w331:dbl)
        n121 = call "disable.vi"("error in (no error)"=w407, "Array"=w401) -> ("error out"=w397:errorcluster)  [unwired: 9 in]
        n122 = call "field_to_voltage_convert.vi"("Start H Field (Oe)"=w382) -> ("Numeric"=w387:dbl)
        n123 = call-poly <vilib>:"DAQmx Write.vi"("task/channels in"=w398, "data"=w387, "error in"=w397) -> ("task out"=w389:refnum<k21>, "error out"=w388:errorcluster)  [unwired: 10 in, 1 out]
        n124 = flat-sequence {
          tunnel: w389 -> [w484]
          tunnel: [w484] -> w381
          tunnel: w388 -> [w483]
          tunnel: [w483] -> w344
          tunnel: w343 -> [w482]
          tunnel: [w482] -> w342
          tunnel: w331 -> [w481]
          frame #0 {
            n125 = Wait (ms)(milliseconds to wait=w481) -> ()  [unwired: 1 out]
          }
        }
        n126 = call <instrlib>:"Send Immediate Trigger.vi"("error in (no error)"=w344, "Channel (1)"=w333, "VISA resource name"=w342) -> ("error out"=w340:errorcluster, "VISA resource name out"=w341:refnum<visa-resource-name>)  [unwired: 7 in]
        n127 = while {
          shift-right: [w414] -> w339
          shift-left: w340 -> [w415]
          shift-right: [w411] -> w338
          shift-left: w341 -> [w412]
          stop <- w413 stop-if-true
          n128 = call <instrlib>:"Query Sweep Complete.vi"("error in (no error)"=w415, "VISA resource name"=w412) -> ("error out"=w414:errorcluster, "Sweep Complete"=w413:bool, "VISA resource name out"=w411:refnum<visa-resource-name>)  [unwired: 7 in]
          n129 = Wait (ms)(milliseconds to wait=u32 1) -> ()  [unwired: 1 out]
        }
        n130 = call <instrlib>:"Read Data.vi"("error in (no error)"=w339, "Data Type (0: FDATA)"=w332, "Channel (1)"=w333, "VISA resource name"=w338) -> ("error out"=w336:errorcluster, "Data"=w337:dbl[], "VISA resource name out"=w335:refnum<visa-resource-name>)  [unwired: 5 in]
        n131 = Add Array Elements(numeric array=w337) -> (sum=w393:dbl)
        n132 = Array Size(array=w337) -> (size(s)=w392:i32)
        n133 = Divide(x=w393, y=w392) -> (x/y=w384:dbl)
        n134 = Unbundle By Name(w367) -> ("Signal"=w385:dbl[], "Field"=w383:dbl[])
        n135 = Build Array (concatenate)(w385, w384) -> (w366:dbl[])
        n136 = Build Array (concatenate)(w383, w382) -> (w365:dbl[])
        n137 = Bundle By Name(cluster=w367, "Signal"=w366, "Field"=w365) -> (w362:T2)
        n138 = Unbundle By Name(w362) -> ("Field"=w361:dbl[], "Signal"=w360:dbl[], "Old Field"=w359:dbl[], "Old Signal"=w358:dbl[])
        n139 = case shown="False" w352 {
          tunnel: [State."Running" w467] -> w370
          tunnel: w381 -> [w454 w457]
          tunnel: [w454 w456] -> w379
          tunnel: w335 -> [w453 w459]
          tunnel: [w453 w458] -> w377
          tunnel: w336 -> [w452 w461]
          tunnel: [w452 w460] -> w376
          tunnel: w380 -> [w451 w466]
          tunnel: [w449 w464] -> w372
          tunnel: w362 -> [w448 w463]
          tunnel: [w448 w462] -> w364
          tunnel: w351 -> [_ w465]
          frame False {
            n140 = Add(x=w451, y=1) -> (x+y=w449:i32)
          }
          frame True {
            n141 = case shown="True" w465 {
              tunnel: [State."Sweeping down" State."Running down"] -> w467
              tunnel: w466 -> [w472 _]
              tunnel: [w472 0] -> w464
              tunnel: w463 -> [w471 w477]
              tunnel: [w471 w477] -> w462
              tunnel: w461 -> [w470 w475]
              tunnel: [w470 w475] -> w460
              tunnel: w459 -> [w469 w478]
              tunnel: [w469 w478] -> w458
              tunnel: w457 -> [w468 w479]
              tunnel: [w468 w479] -> w456
              frame False {
              }
              frame True {
                n142 = Wait (ms)(milliseconds to wait=u32 5000) -> ()  [unwired: 1 out]
              }
            }
          }
        }
        n143 = Bundle("Field"=w361, "Signal"=w360) -> (w357:cluster{"Field":dbl[], "Signal":dbl[]})  [unwired: 1 in]
        n144 = Bundle("Old Field"=w359, "Old Signal"=w358) -> (w356:cluster{"Old Field":dbl[], "Old Signal":dbl[]})  [unwired: 1 in]
        n145 = Build Array(w357, w356) -> (w350:cluster{"Old Field":dbl[], "Old Signal":dbl[]}[])
        n146 = case shown="False" w374 {
          tunnel: [w437 w446] -> w369
          tunnel: w379 -> [w436 w445]
          tunnel: [w436 w445] -> w378
          tunnel: w377 -> [w435 w444]
          tunnel: [w435 w444] -> w334
          tunnel: w376 -> [w434 w443]
          tunnel: [w434 w443] -> w375
          tunnel: w373 -> [w433 w442]
          tunnel: w372 -> [w432 w441]
          tunnel: [w432 w441] -> w371
          tunnel: w370 -> [w430 _]
          tunnel: [w431 w440] -> w363
          tunnel: w364 -> [w431 w440]
          frame False {
            n147 = Or(x=w434, y=w433) -> (x .or. y?=w438:bool)
            n148 = call "error_check_shutdown_sweep_field.vi"("State In"=w430, "Boolean"=w438) -> ("State Out"=w437:T1)  [unwired: 9 in]
          }
          frame True {
            n149 = Or(x=w443, y=w442) -> (x .or. y?=w447:bool)
            n150 = call "error_check_shutdown_sweep_field.vi"("State In"=State."Sweeping down", "Boolean"=w447) -> ("State Out"=w446:T1)  [unwired: 9 in]
          }
        }
      }
      frame "Running down" {
        (unwired) 0
        # "field step"
        # "averaging"
        n151 = control-ref of="Status"() -> (w557:refnum<vi>)
        n152 = Subtract(x=w508, y=w509) -> (x-y=w515:dbl)
        n153 = Subtract(x=w512, y=1) -> (x-y=w517:i32)
        n154 = case shown="1" w489 {
          tunnel: [2 ("Channel (1)") 1 ("Channel (1)")] -> w488
          tunnel: ["Meas_S11" ("Measurement Name (CH1_S11_1)") "Meas_S21" ("Measurement Name (CH1_S11_1)")] -> _
          frame 0, Default {
          }
          frame 1 {
          }
        }
        n155 = call "change_status.vi"("error in (no error)"=w558, "String"="Measurement running...", "String in"=w557) -> ("error out"=w559:errorcluster)  [unwired: 8 in]
        n156 = Divide(x=w515, y=w517) -> (x/y=w500:dbl)
        n157 = Greater Or Equal?(x=w508, y=w509) -> (x >= y?=w514:bool)
        n158 = call "enable.vi"("error in (no error)"=w559, "Array"=w555) -> ("error out"=w562:errorcluster)  [unwired: 9 in]
        n159 = Absolute Value(x=w500) -> (abs(x)=w499:dbl)
        n160 = Divide(x=w499, y=w501) -> (x/y=w504:dbl)
        n161 = call "disable.vi"("error in (no error)"=w562, "Array"=w554) -> ("error out"=w561:errorcluster)  [unwired: 9 in]
        n162 = Multiply(x=w513, y=w500) -> (x*y=w516:dbl)
        n163 = Multiply(x=w504, y=1000.0) -> (x*y=w502:dbl)
        n164 = call "disable.vi"("error in (no error)"=w561, "Array"=w553) -> ("error out"=w560:errorcluster)  [unwired: 9 in]
        n165 = case shown="True" w514 {
          tunnel: w516 -> [w577 w582]
          tunnel: [w576 w580] -> w510
          tunnel: [w575 w581] -> w511
          tunnel: w509 -> [w574 w578]
          tunnel: w508 -> [w573 w579]
          frame False {
            n166 = Add(x=w574, y=w577) -> (x+y=w576:dbl)
            n167 = Less Or Equal?(x=w576, y=w573) -> (x <= y?=w575:bool)
          }
          frame True {
            n168 = Add(x=w578, y=w582) -> (x+y=w580:dbl)
            n169 = Greater Or Equal?(x=w580, y=w579) -> (x >= y?=w581:bool)
          }
        }
        n170 = call "disable.vi"("error in (no error)"=w560, "Array"=w552) -> ("error out"=w533:errorcluster)  [unwired: 9 in]
        n171 = call "field_to_voltage_convert.vi"("Start H Field (Oe)"=w510) -> ("Numeric"=w506:dbl)
        n172 = call-poly <vilib>:"DAQmx Write.vi"("task/channels in"=w532, "data"=w506, "error in"=w533) -> ("task out"=w549:refnum<k21>, "error out"=w548:errorcluster)  [unwired: 10 in, 1 out]
        n173 = flat-sequence {
          tunnel: w502 -> [w618]
          tunnel: w549 -> [w617]
          tunnel: [w617] -> w544
          tunnel: w548 -> [w616]
          tunnel: [w616] -> w490
          tunnel: w498 -> [w615]
          tunnel: [w615] -> w492
          frame #0 {
            n174 = Wait (ms)(milliseconds to wait=w618) -> ()  [unwired: 1 out]
          }
        }
        n175 = call <instrlib>:"Send Immediate Trigger.vi"("error in (no error)"=w490, "Channel (1)"=w488, "VISA resource name"=w492) -> ("error out"=w495:errorcluster, "VISA resource name out"=w496:refnum<visa-resource-name>)  [unwired: 7 in]
        n176 = while {
          shift-right: [w571] -> w494
          shift-left: w495 -> [w572]
          shift-right: [w568] -> w493
          shift-left: w496 -> [w569]
          stop <- w570 stop-if-true
          n177 = call <instrlib>:"Query Sweep Complete.vi"("error in (no error)"=w572, "VISA resource name"=w569) -> ("error out"=w571:errorcluster, "Sweep Complete"=w570:bool, "VISA resource name out"=w568:refnum<visa-resource-name>)  [unwired: 7 in]
          n178 = Wait (ms)(milliseconds to wait=u32 1) -> ()  [unwired: 1 out]
        }
        n179 = call <instrlib>:"Read Data.vi"("error in (no error)"=w494, "Data Type (0: FDATA)"=w487, "Channel (1)"=w488, "VISA resource name"=w493) -> ("error out"=w486:errorcluster, "Data"=w485:dbl[], "VISA resource name out"=w491:refnum<visa-resource-name>)  [unwired: 5 in]
        n180 = Add Array Elements(numeric array=w485) -> (sum=w551:dbl)
        n181 = Array Size(array=w485) -> (size(s)=w550:i32)
        n182 = Divide(x=w551, y=w550) -> (x/y=w546:dbl)
        n183 = Unbundle By Name(w530) -> ("Signal"=w547:dbl[], "Field"=w545:dbl[])
        n184 = Build Array (concatenate)(w547, w546) -> (w538:dbl[])
        n185 = Build Array (concatenate)(w545, w510) -> (w537:dbl[])
        n186 = Bundle By Name(cluster=w530, "Signal"=w538, "Field"=w537) -> (w535:T2)
        n187 = Unbundle By Name(w535) -> ("Field"=w525:dbl[], "Signal"=w526:dbl[], "Old Field"=w527:dbl[], "Old Signal"=w528:dbl[])
        n188 = case shown="False" w511 {
          tunnel: [State."Running down" State."Sweeping down"] -> w539
          tunnel: w544 -> [w607 w612]
          tunnel: [w607 w612] -> w543
          tunnel: w491 -> [w606 w613]
          tunnel: [w606 w613] -> w542
          tunnel: w486 -> [w605 w611]
          tunnel: [w605 w611] -> w541
          tunnel: w513 -> [w604 w609]
          tunnel: [w602 w609] -> w540
          tunnel: w535 -> [w601 w610]
          tunnel: [w601 w610] -> w536
          frame False {
            n189 = Add(x=w604, y=1) -> (x+y=w602:i32)
          }
          frame True {
          }
        }
        n190 = Bundle("Field"=w525, "Signal"=w526) -> (w534:cluster{"Field":dbl[], "Signal":dbl[]})  [unwired: 1 in]
        n191 = Bundle("Old Field"=w527, "Old Signal"=w528) -> (w529:cluster{"Old Field":dbl[], "Old Signal":dbl[]})  [unwired: 1 in]
        n192 = Build Array(w534, w529) -> (w507:cluster{"Old Field":dbl[], "Old Signal":dbl[]}[])
        n193 = case shown="False" w531 {
          tunnel: [w590 w599] -> w519
          tunnel: w543 -> [w589 w598]
          tunnel: [w589 w598] -> w520
          tunnel: w542 -> [w588 w597]
          tunnel: [w588 w597] -> w497
          tunnel: w541 -> [w587 w596]
          tunnel: [w587 w596] -> w521
          tunnel: w524 -> [w586 w595]
          tunnel: w540 -> [w585 w594]
          tunnel: [w585 w594] -> w522
          tunnel: w539 -> [w583 _]
          tunnel: [w584 w593] -> w523
          tunnel: w536 -> [w584 w593]
          frame False {
            n194 = Or(x=w587, y=w586) -> (x .or. y?=w591:bool)
            n195 = call "error_check_shutdown_sweep_field.vi"("State In"=w583, "Boolean"=w591) -> ("State Out"=w590:T1)  [unwired: 9 in]
          }
          frame True {
            n196 = Or(x=w596, y=w595) -> (x .or. y?=w600:bool)
            n197 = call "error_check_shutdown_sweep_field.vi"("State In"=State."Sweeping down", "Boolean"=w600) -> ("State Out"=w599:T1)  [unwired: 9 in]
          }
        }
      }
      frame "Shutdown" {
        w639 = T3 1 items=["no dialog", "OK message", "continue or stop message", "OK message + warnings", "continue/stop + warnings"] ("type of dialog (OK msg:1)")
        n198 = control-ref of="Status"() -> (w644:refnum<vi>)
        n199 = call "change_status.vi"("error in (no error)"=w643, "String"="Shutting down...Sweeping field to zero...", "String in"=w644) -> ("error out"=w650:errorcluster)  [unwired: 8 in]
        n200 = call "disable.vi"("error in (no error)"=w650, "Array"=w648) -> ("error out"=w653:errorcluster)  [unwired: 9 in]
        n201 = Wait (ms)(milliseconds to wait=u32 1000) -> ()  [unwired: 1 out]
        n202 = call "disable.vi"("error in (no error)"=w653, "Array"=w647) -> ("error out"=w652:errorcluster)  [unwired: 9 in]
        n203 = call "disable.vi"("error in (no error)"=w652, "Array"=w646) -> ("error out"=w651:errorcluster)  [unwired: 9 in]
        n204 = call "disable.vi"("error in (no error)"=w651, "Array"=w645) -> ("error out"=w635:errorcluster)  [unwired: 9 in]
        n205 = call-poly <vilib>:"DAQmx Write.vi"("task/channels in"=w634, "data"=0.0, "error in"=w635) -> ("task out"=w632:refnum<k21>, "error out"=w633:errorcluster)  [unwired: 10 in, 1 out]
        n206 = call <vilib>:"DAQmx Stop Task.vi"("task/channels in"=w632, "error in"=w633) -> ("task out"=w641:refnum<k21>, "error out"=w642:errorcluster)  [unwired: 12 in]
        n207 = call <vilib>:"DAQmx Clear Task.vi"("task in"=w641, "error in"=w642) -> ("error out"=w621:errorcluster)  [unwired: 13 in]
        n208 = call <instrlib>:"Abort Sweep.vi"("error in (no error)"=w621, "VISA resource name"=w622) -> ("error out"=w623:errorcluster, "VISA resource name out"=w619:refnum<visa-resource-name>)  [unwired: 8 in]
        n209 = call <instrlib>:"Close.vi"("error in (no error)"=w623, "VISA resource name"=w619) -> ("error out"=w620:errorcluster)  [unwired: 9 in]
        n210 = property on="SpectrumGraph" class="XYGraph (strict)"(error in=w620, "Value"=cluster{"Old Field":dbl[], "Old Signal":dbl[]}[] [] ("SpectrumGraph")) -> (error out=w628:errorcluster)  [unwired: 1 in, 1 out]
        n211 = control-ref of="Status"() -> (w625:refnum<vi>)
        n212 = call "change_status.vi"("error in (no error)"=w628, "String"="Off", "String in"=w625) -> ("error out"=w627:errorcluster)  [unwired: 8 in]
        n213 = call <vilib>:"Simple Error Handler.vi"("type of dialog (OK msg:1)"=w639, "error in (no error)"=w627) -> ("error out"=w640:errorcluster)  [unwired: 3 in, 4 out]
      }
    }
    "SpectrumGraph" <- w48
    n214 = event shown="[0] Timeout" {
      selector: _ -> [_ _ _]
      dyn-events: _ -> [_ _ _]
      timeout: 1 -> [_ _ _]
      event Timeout {
        n215 = event-data() -> ()  [unwired: 1 in, 3 out]
      }
      event "SpectrumGraph": Mouse Down {
        n216 = event-data() -> ("CtlRef"=w83:refnum<vi>, "Coords"=w82:T4)  [unwired: 1 in]
        n217 = invoke on="Invoke Node" class="XYGraph (strict)" method="Map Coords To XY"(reference=w83, "Coords"=w82) -> ("Map Coords To XY"=w84:bool, "XY"=w85:cluster{"X":dbl, "Y":dbl})  [unwired: 5 in, 5 out]
        n218 = case shown="True" w84 {
          tunnel: w85 -> [_ w86]
          frame False {
          }
          frame True {
            n219 = property on="Cursor" class="Clust (strict)"("Value"=w86) -> ()  [unwired: 2 in, 2 out]
          }
        }
      }
      event "Save Button": Value Change {
        # "Field\nSignal"
        n220 = event-data() -> ()  [unwired: 1 in, 1 out]
        n221 = control-ref of="SpectrumGraph"() -> (w95:refnum<vi>)
        n222 = property class="XYGraph (strict)"(reference=w95) -> ("Value"=w93:cluster{"Old Field":dbl[], "Old Signal":dbl[]}[])  [unwired: 1 in, 2 out]
        n223 = Index Array(array=w93, index=1) -> (element=w92:cluster{"Old Field":dbl[], "Old Signal":dbl[]})
        n224 = Unbundle(w92) -> ("Old Field"=w88:dbl[], "Old Signal"=w87:dbl[])
        n225 = call "Convert to Dynamic Data"("Array"=w88) -> ("Dynamic Data Type"=w91:dynamicdata)  [unwired: 3 in]
        n226 = call "Convert to Dynamic Data2"("Array"=w87) -> ("Dynamic Data Type"=w90:dynamicdata)  [unwired: 3 in]
        n227 = Merge Signals(w91, w90) -> (w89:dynamicdata)
        n228 = call "Write To Measurement File"("Signals"=w89) -> ()  [unwired: 16 in, 3 out]
      }
    }
    n229 = case shown="False" "Clear button" {
      tunnel: w46 -> [w77 w81]
      tunnel: [w77 w80] -> w45
      frame False {
      }
      frame True {
        n230 = Bundle By Name(cluster=w81, "Old Field"=dbl[] [], "Old Signal"=dbl[] []) -> (w80:T2)
      }
    }
  }
  "Error Out" <- w12
  "DAQ channel Out" <- w17
  "Analyzer Name Out" <- w8
  "Cursor" <- cluster{"x":dbl, "y":dbl} {"x"=0.0, "y"=0.0} ("Cursor")
